vi "Control Panel.vi"(8 "error in (no error)":errorcluster, 11 "Fake Microwave in":refnum<class "Microwave.lvclass">) -> (0 "error out":errorcluster, 3 "Fake Microwave out":refnum<class "Microwave.lvclass">)   [LabVIEW 2023, in "Microwave.lvclass"]
uses:
  Microwave.lvclass
  Microwave.lvclass/Microwave.ctl
  Utility Classes/Scannable/Scannable.lvclass
  Agilent PSG MXG Series/Agilent PSG MXG Series.lvlib
panel:
  out "Ready when blinking":bool
  out "Amplitude Mode":enum16{"Fixed", "Stepped Sweep", "List Sweep"}(ring)
  out "Frequency Mode":T1(ring)
  in  "Amplitude Mode Set":enum16{"Fixed", "Stepped Sweep", "List Sweep"}(ring)
  in  "Frequency Mode Set":T1(ring)
  in  "Copy actual to set":bool
  in  "Populate fields with member data":bool
  out "Dwell":dbl[unit]
  out "Points":i32
  in  "Dwell Set":dbl[unit]
  in  "Points Set":i32
  out "Freq Stop":dbl[unit]
  out "Freq Start":dbl[unit]
  in  "Freq Stop Set":dbl[unit]
  in  "Freq Start Set":dbl[unit]
  out "Amp Stop":dbl
  out "Amp Start":dbl
  in  "Amp Stop Set":dbl
  in  "Amp Start Set":dbl
  out "Amplitude":dbl
  out "Frequency":dbl[unit]
  in  "Amplitude Set":dbl
  in  "Frequency Set":dbl[unit]
  in  "Rf On/Off":bool caption="rf On/Off"
  in  "Exit":bool
  in  "Set":bool
  in  "Read to Control":bool
  in  "Read":bool
  in  "Reset":bool
  # "Microwave Front Panel"
  # "Output Mode"
  # "CW Operation Settings"
  # "Generic Sweep Settings"
  # "dBm"
  # "dBm"
  # "Frequency Sweep Settings"
  # "Amplitude Sweep Settings"
  # "dBm"
  # "dBm"
  # "dBm"
  # "dBm"
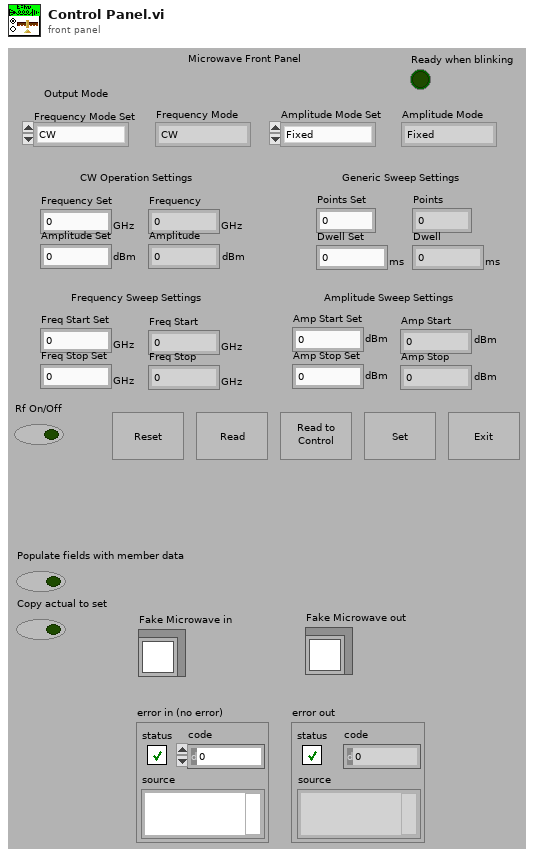
[diagram p1: front panel]
types:
  T1 = enum16{"CW", "Fixed", "Stepped Sweep", "List Sweep"}
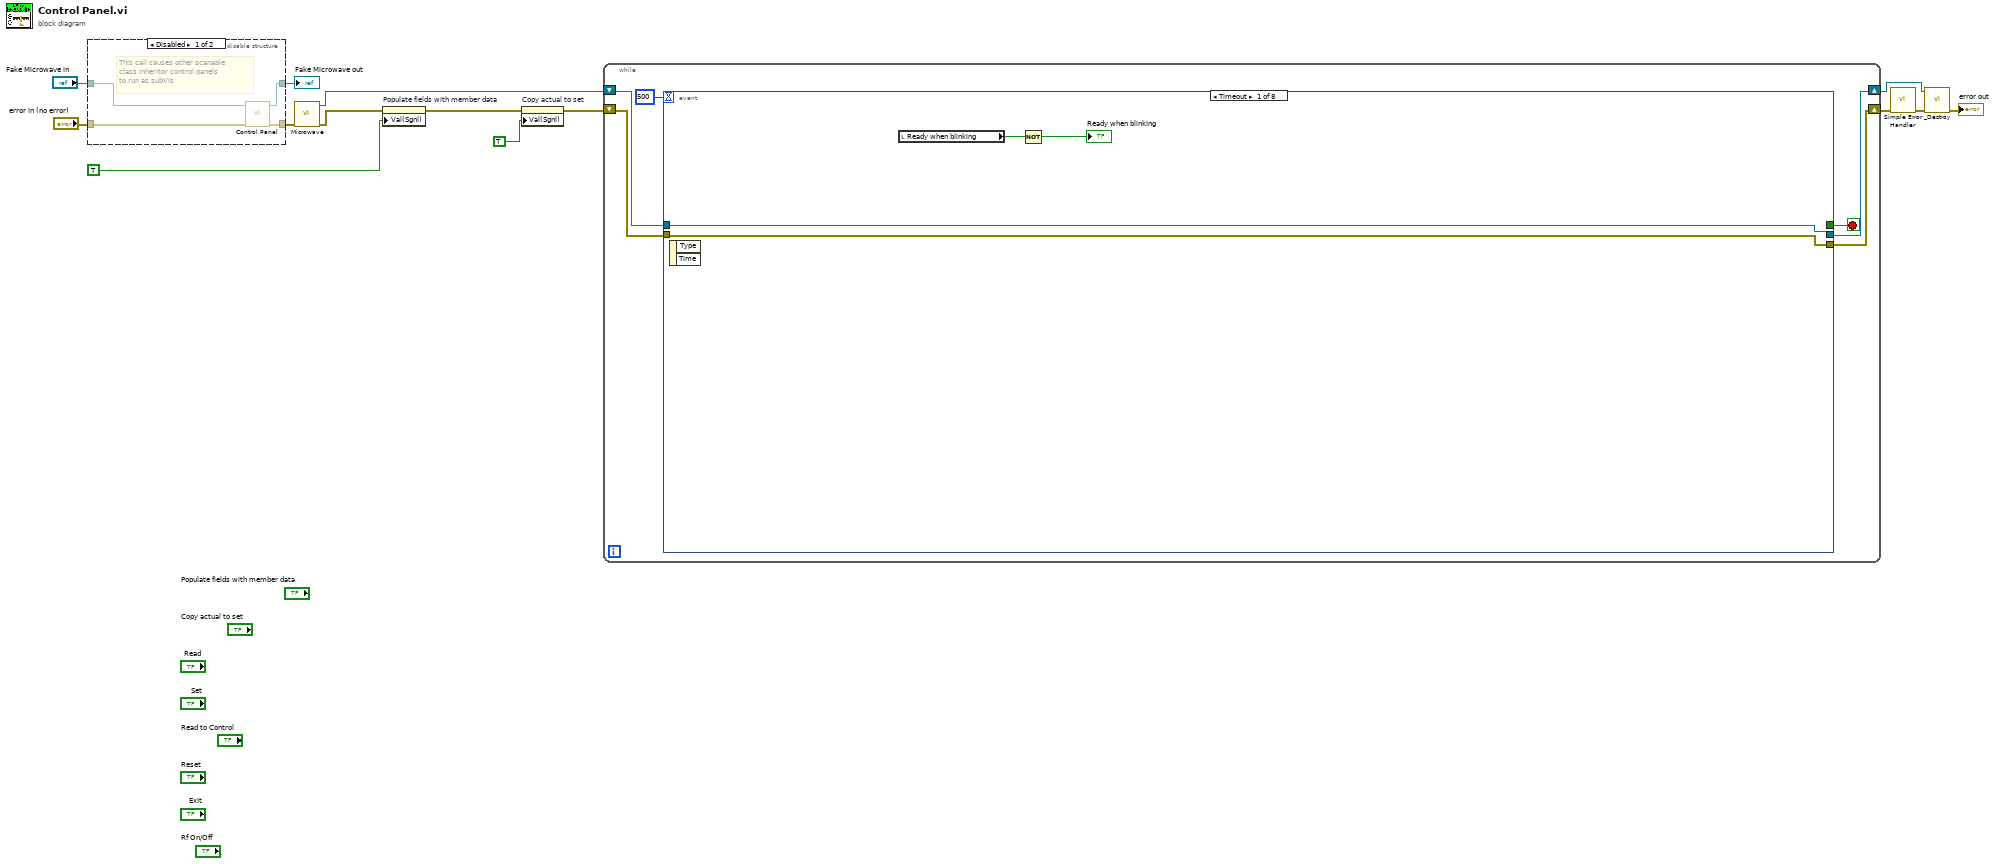
[diagram p0: block diagram]
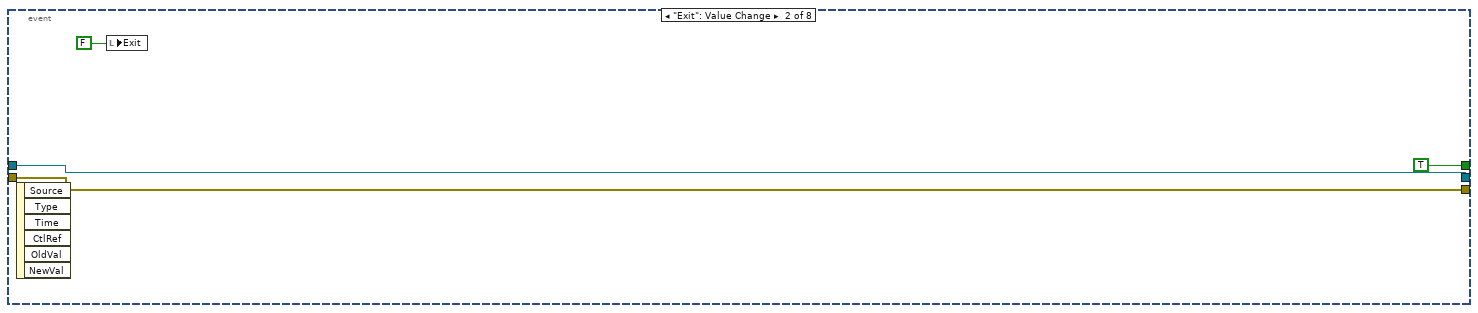
[diagram p3: hidden frame]
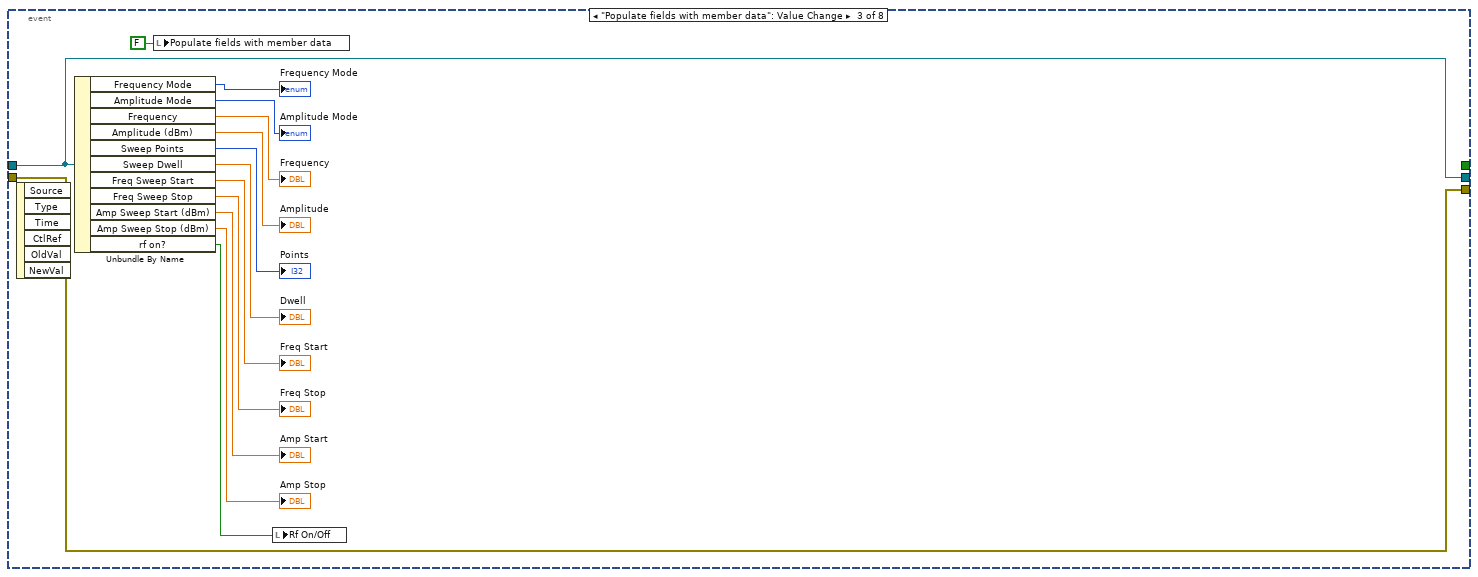
[diagram p4: hidden frame]
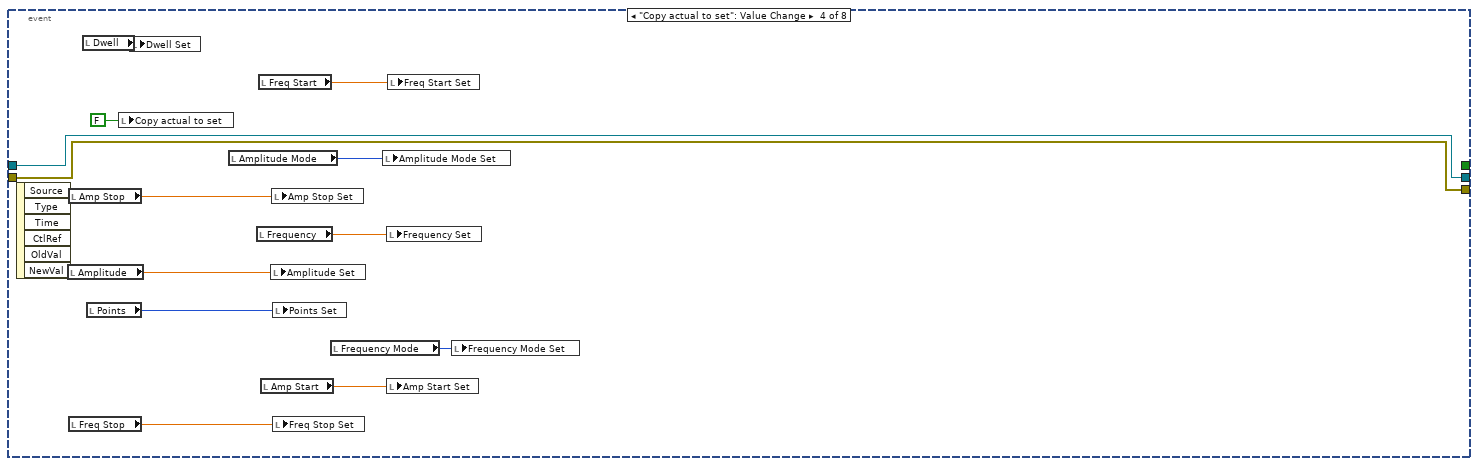
[diagram p5: hidden frame]
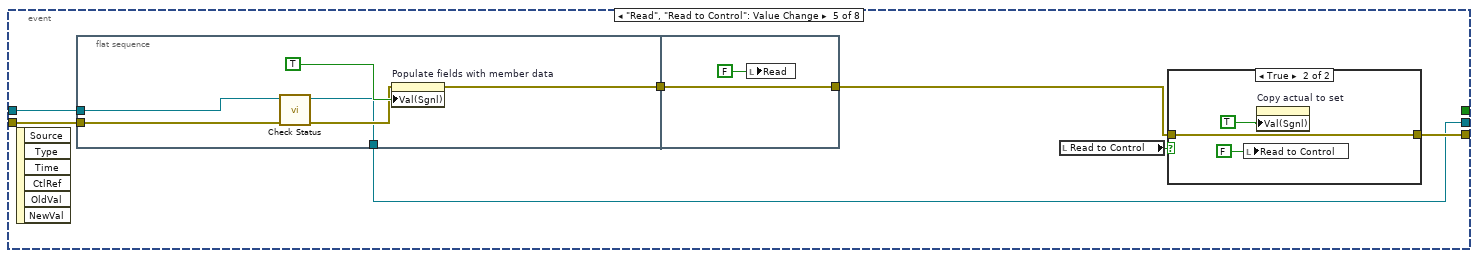
[diagram p6: hidden frame]
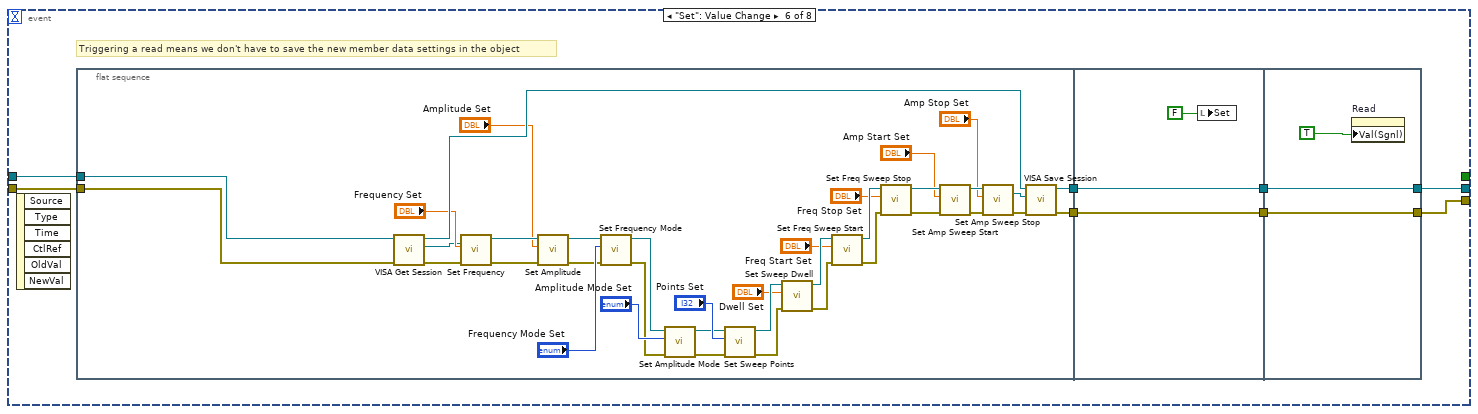
[diagram p8: hidden frame]
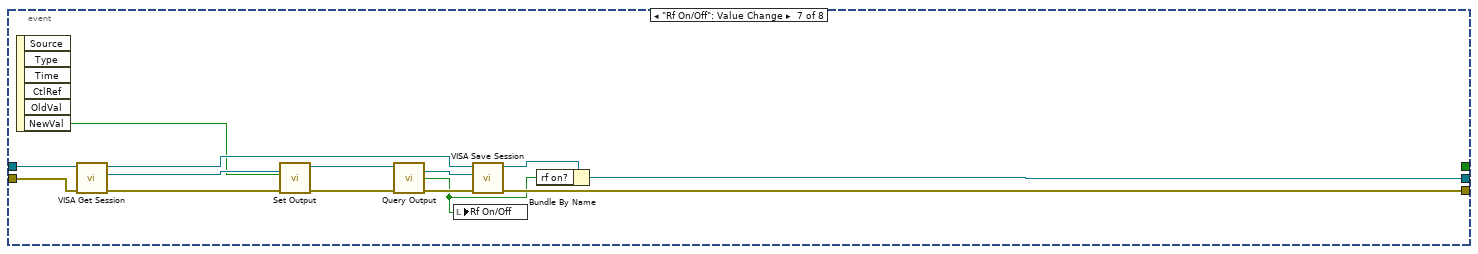
[diagram p9: hidden frame]
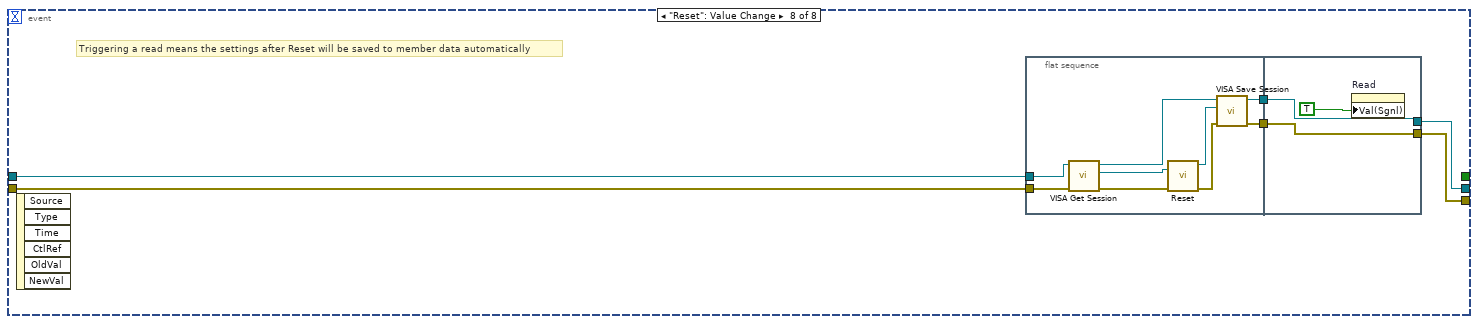
[diagram p10: hidden frame]
diagram:
  n1 = disable-structure shown="Disabled" {
    disable-tunnel: "error in (no error)" -> [w18 w19]
    disable-tunnel: "Fake Microwave in" -> [w17 w20]
    disable-tunnel: [w16 w19] -> w10
    disable-tunnel: [w15 w20] -> w9
    frame Disabled {
      # "This call causes other scanable\nclass inheritor control panels\nto run as subVIs"
      n2 = call-parent "Control Panel.vi"("error in (no error)"=w18, "Instrument in"=w17) -> ("error out"=w16:errorcluster, "Instrument out"=w15:refnum<class "Microwave.lvclass">)  [unwired: 8 out]
    }
    frame Enabled {
    }
  }
  "Fake Microwave out" <- w9
  n3 = call "Microwave.vi"("error in (no error)"=w10) -> ("error out"=w11:errorcluster, "Microwave out"=w3:refnum<class "Microwave.lvclass">)  [unwired: 9 out]
  n4 = property on="Populate fields with member data" class="Bool (strict)"(error in=w11, "Val(Sgnl)"=TRUE ("Value (Signaling)")) -> (error out=w7:errorcluster)  [unwired: 1 in, 1 out]
  n5 = property on="Copy actual to set" class="Bool (strict)"(error in=w7, "Val(Sgnl)"=TRUE ("Value (Signaling)")) -> (error out=w1:errorcluster)  [unwired: 1 in, 1 out]
  n6 = while {
    shift-right: [w24] -> w4
    shift-left: w1 -> [w23]
    shift-right: [w25] -> w2
    shift-left: w3 -> [w26]
    stop <- w22 stop-if-true
    n7 = event shown="[0] Timeout" {
      selector: _ -> [_ _ _ _ _ _ _ _]
      dyn-events: _ -> [_ _ _ _ _ _ _ _]
      timeout: 500 -> [_ _ _ _ _ _ _ _]
      tunnel: w26 -> [w30 w34 w37 w61 w63 w88 w145 w151]
      tunnel: [w30 w34 w37 w61 w62 w87 w138 w150] -> w25
      tunnel: [w29 w33 w48 w60 w64 w85 w143 w148] -> w24
      tunnel: w23 -> [w29 w33 w48 w60 w67 w86 w144 w149]
      tunnel: [_ TRUE ("exit") _ _ _ _ _ _] -> w22
      event Timeout {
        n8 = event-data() -> ()  [unwired: 3 out]
        n9 = local read "Ready when blinking"() -> (w27:bool)
        n10 = Not(x=w27) -> (.not. x?=→"Ready when blinking":bool)
      }
      event "Exit": Value Change {
        n11 = event-data() -> ()  [unwired: 7 out]
        n12 = local write "Exit"(FALSE ("Exit")) -> ()
      }
      event "Populate fields with member data": Value Change {
        n13 = event-data() -> ()  [unwired: 7 out]
        n14 = Unbundle By Name(w37) -> ("Frequency Mode"=→"Frequency Mode":u16, "Amplitude Mode"=→"Amplitude Mode":u16, "Frequency"=→"Frequency":dbl[unit], "Amplitude (dBm)"=→"Amplitude":dbl, "Sweep Points"=→"Points":i32, "Sweep Dwell"=→"Dwell":dbl[unit], "Freq Sweep Start"=→"Freq Start":dbl[unit], "Freq Sweep Stop"=→"Freq Stop":dbl[unit], "Amp Sweep Start (dBm)"=→"Amp Start":dbl, "Amp Sweep Stop (dBm)"=→"Amp Stop":dbl, "rf on?"=w35:bool)
        n15 = local write "Populate fields with member data"(FALSE ("Populate fields with member data")) -> ()
        n16 = local write "Rf On/Off"(w35) -> ()
      }
      event "Copy actual to set": Value Change {
        n17 = event-data() -> ()  [unwired: 7 out]
        n18 = local read "Amplitude"() -> (w56:dbl)
        n19 = local read "Amp Stop"() -> (w50:dbl)
        n20 = local read "Freq Stop"() -> (w52:dbl[unit])
        n21 = local read "Dwell"() -> (w54:dbl[unit])
        n22 = local read "Points"() -> (w55:i32)
        n23 = local write "Copy actual to set"(FALSE ("Copy actual to set")) -> ()
        n24 = local write "Dwell Set"(w54) -> ()
        n25 = local read "Amplitude Mode"() -> (w58:enum16{"Fixed", "Stepped Sweep", "List Sweep"})
        n26 = local read "Frequency"() -> (w57:dbl[unit])
        n27 = local read "Freq Start"() -> (w53:dbl[unit])
        n28 = local read "Amp Start"() -> (w51:dbl)
        n29 = local write "Amplitude Set"(w56) -> ()
        n30 = local write "Amp Stop Set"(w50) -> ()
        n31 = local write "Points Set"(w55) -> ()
        n32 = local write "Freq Stop Set"(w52) -> ()
        n33 = local read "Frequency Mode"() -> (w59:T1)
        n34 = local write "Amplitude Mode Set"(w58) -> ()
        n35 = local write "Frequency Set"(w57) -> ()
        n36 = local write "Amp Start Set"(w51) -> ()
        n37 = local write "Freq Start Set"(w53) -> ()
        n38 = local write "Frequency Mode Set"(w59) -> ()
      }
      event "Read", "Read to Control": Value Change {
        n39 = event-data() -> ()  [unwired: 7 out]
        n40 = flat-sequence {
          tunnel: w63 -> [w78]
          tunnel: w67 -> [w77]
          tunnel: [w74] -> w65
          tunnel: [w73] -> w62
          tunnel: [w79] -> w66
          tunnel: w65 -> [w79]
          frame #0 {
            n41 = call-dynamic "Check Status.vi"("error in (no error)"=w77, "Microwave in"=w78) -> ("error out"=w75:errorcluster, "Microwave out"=w73:refnum<class "Microwave.lvclass">)  [unwired: 8 out]
            n42 = property on="Populate fields with member data" class="Bool (strict)"(error in=w75, "Val(Sgnl)"=TRUE ("Value (Signaling)")) -> (error out=w74:errorcluster)  [unwired: 1 in, 1 out]
          }
          frame #1 {
            n43 = local write "Read"(FALSE ("Read")) -> ()
          }
        }
        n44 = local read "Read to Control"() -> (w68:bool)
        n45 = case shown="True" w68 {
          tunnel: [w69 w72] -> w64
          tunnel: w66 -> [w69 w72]
          frame False {
          }
          frame True {
            n46 = local write "Read to Control"(FALSE ("Read to Control")) -> ()
            n47 = property on="Copy actual to set" class="Bool (strict)"("Val(Sgnl)"=TRUE ("Value (Signaling)")) -> ()  [unwired: 2 in, 2 out]
          }
        }
      }
      event "Set": Value Change {
        # "Triggering a read means we don't have to save the new member data settings in the object"
        n48 = event-data() -> ()  [unwired: 7 out]
        n49 = flat-sequence {
          tunnel: w88 -> [w124]
          tunnel: w86 -> [w122]
          tunnel: [w123] -> w84
          tunnel: [w121] -> w83
          tunnel: w84 -> [w128]
          tunnel: w83 -> [w127]
          tunnel: [w128] -> w82
          tunnel: [w127] -> w81
          tunnel: [w130] -> w85
          tunnel: [w131] -> w87
          tunnel: w82 -> [w131]
          tunnel: w81 -> [w130]
          frame #0 {
            n50 = call-dynamic "VISA Get Session.vi"("error in (no error)"=w122, "Instrument.lvclass in"=w124) -> ("error out"=w92:errorcluster, "VISA Resource Name"=w94:refnum<visa-resource-name>, "Instrument.lvclass out"=w125:refnum<class "Microwave.lvclass">)  [unwired: 7 out]
            n51 = call "Set Frequency.vi"("error in (no error)"=w92, "Frequency"="Frequency Set", "VISA resource name"=w94) -> ("error out"=w112:errorcluster, "VISA resource name out"=w119:refnum<visa-resource-name>)  [unwired: 7 out]
            n52 = call "Set Amplitude.vi"("error in (no error)"=w112, "Amplitude (dBm)"="Amplitude Set", "VISA resource name"=w119) -> ("error out"=w91:errorcluster, "VISA resource name out"=w93:refnum<visa-resource-name>)  [unwired: 7 out]
            n53 = call "Set Frequency Mode.vi"("error in (no error)"=w91, "Frequency Mode"="Frequency Mode Set", "VISA resource name"=w93) -> ("error out"=w95:errorcluster, "VISA resource name out"=w120:refnum<visa-resource-name>)  [unwired: 7 out]
            n54 = call "Set Amplitude Mode.vi"("error in (no error)"=w95, "Amplitude Mode"="Amplitude Mode Set", "VISA resource name"=w120) -> ("error out"=w90:errorcluster, "VISA resource name out"=w89:refnum<visa-resource-name>)  [unwired: 7 out]
            n55 = call "Set Sweep Points.vi"("error in (no error)"=w90, "Number of Sweep Points"="Points Set", "VISA resource name"=w89) -> ("error out"=w111:errorcluster, "VISA resource name out"=w118:refnum<visa-resource-name>)  [unwired: 7 out]
            n56 = call "Set Sweep Dwell.vi"("error in (no error)"=w111, "Sweep Dwell Time"="Dwell Set", "VISA resource name"=w118) -> ("error out"=w110:errorcluster, "VISA resource name out"=w117:refnum<visa-resource-name>)  [unwired: 7 out]
            n57 = call "Set Freq Sweep Start.vi"("error in (no error)"=w110, "Frequency Sweep Start"="Freq Start Set", "VISA resource name"=w117) -> ("error out"=w109:errorcluster, "VISA resource name out"=w116:refnum<visa-resource-name>)  [unwired: 7 out]
            n58 = call "Set Freq Sweep Stop.vi"("error in (no error)"=w109, "Frequency Sweep Stop"="Freq Stop Set", "VISA resource name"=w116) -> ("error out"=w108:errorcluster, "VISA resource name out"=w115:refnum<visa-resource-name>)  [unwired: 7 out]
            n59 = call "Set Amp Sweep Start.vi"("error in (no error)"=w108, "Amplitude Sweep Start (dBm)"="Amp Start Set", "VISA resource name"=w115) -> ("error out"=w107:errorcluster, "VISA resource name out"=w114:refnum<visa-resource-name>)  [unwired: 7 out]
            n60 = call "Set Amp Sweep Stop.vi"("error in (no error)"=w107, "Amplitude Sweep Stop (dBm)"="Amp Stop Set", "VISA resource name"=w114) -> ("error out"=w106:errorcluster, "VISA resource name out"=w113:refnum<visa-resource-name>)  [unwired: 7 out]
            n61 = call-dynamic "VISA Save Session.vi"("error in (no error)"=w106, "VISA Resource Name"=w113, "Instrument.lvclass in"=w125) -> ("error out"=w121:errorcluster, "Instrument.lvclass out"=w123:refnum<class "Microwave.lvclass">)  [unwired: 7 out]
          }
          frame #1 {
            n62 = local write "Set"(FALSE ("Set")) -> ()
          }
          frame #2 {
            n63 = property on="Read" class="Bool (strict)"("Val(Sgnl)"=TRUE ("Value (Signaling)")) -> ()  [unwired: 2 in, 2 out]
          }
        }
      }
      event "Rf On/Off": Value Change {
        n64 = event-data() -> ("NewVal"=w137:bool)  [unwired: 6 out]
        n65 = call-dynamic "VISA Get Session.vi"("error in (no error)"=w144, "Instrument.lvclass in"=w145) -> ("error out"=w141:errorcluster, "VISA Resource Name"=w142:refnum<visa-resource-name>, "Instrument.lvclass out"=w140:refnum<class "Microwave.lvclass">)  [unwired: 7 out]
        n66 = call "Set Output.vi"("error in (no error)"=w141, "Output On"=w137, "VISA resource name"=w142) -> ("error out"=w134:errorcluster, "VISA resource name out"=w136:refnum<visa-resource-name>)  [unwired: 7 out]
        n67 = call "Query Output.vi"("error in (no error)"=w134, "VISA resource name"=w136) -> ("error out"=w133:errorcluster, "Output On?"=w132:bool, "VISA resource name out"=w135:refnum<visa-resource-name>)  [unwired: 7 out]
        n68 = local write "Rf On/Off"(w132) -> ()
        n69 = call-dynamic "VISA Save Session.vi"("error in (no error)"=w133, "VISA Resource Name"=w135, "Instrument.lvclass in"=w140) -> ("error out"=w143:errorcluster, "Instrument.lvclass out"=w139:refnum<class "Microwave.lvclass">)  [unwired: 7 out]
        n70 = Bundle By Name(cluster=w139, "rf on?"=w132) -> (w138:refnum<class "Microwave.lvclass">)
      }
      event "Reset": Value Change {
        # "Triggering a read means the settings after Reset will be saved to member data automatically"
        n71 = event-data() -> ()  [unwired: 7 out]
        n72 = flat-sequence {
          tunnel: w151 -> [w155]
          tunnel: w149 -> [w153]
          tunnel: [w154] -> w147
          tunnel: [w152] -> w146
          tunnel: [w162] -> w148
          tunnel: [w163] -> w150
          tunnel: w147 -> [w163]
          tunnel: w146 -> [w162]
          frame #0 {
            n73 = call-dynamic "VISA Get Session.vi"("error in (no error)"=w153, "Instrument.lvclass in"=w155) -> ("error out"=w158:errorcluster, "VISA Resource Name"=w160:refnum<visa-resource-name>, "Instrument.lvclass out"=w159:refnum<class "Microwave.lvclass">)  [unwired: 7 out]
            n74 = call "Reset.vi"("error in (no error)"=w158, "VISA resource name"=w160) -> ("error out"=w157:errorcluster, "VISA resource name out"=w156:refnum<visa-resource-name>)  [unwired: 8 out]
            n75 = call-dynamic "VISA Save Session.vi"("error in (no error)"=w157, "VISA Resource Name"=w156, "Instrument.lvclass in"=w159) -> ("error out"=w152:errorcluster, "Instrument.lvclass out"=w154:refnum<class "Microwave.lvclass">)  [unwired: 7 out]
          }
          frame #1 {
            n76 = property on="Read" class="Bool (strict)"("Val(Sgnl)"=TRUE ("Value (Signaling)")) -> ()  [unwired: 2 in, 2 out]
          }
        }
      }
    }
  }
  n77 = call <vilib>:"Simple Error Handler.vi"("error in (no error)"=w4) -> ("error out"=w6:errorcluster)  [unwired: 1 in, 7 out]
  n78 = call-dynamic "_Destroy.vi"("error in (no error)"=w6, "Instrument in"=w2) -> ("error out"=→"error out":errorcluster)  [unwired: 9 out]
